vi "PXI_Health_Loop.vi"(8 "error in (no error)":errorcluster) -> (0 "error out":errorcluster)   [LabVIEW 2018]
uses:
  Controls/Enums/PXI_Loop_Enum.ctl
  Controls/Clusts/PXI_Health.ctl
  Controls/Enums/FP_Loop_Enum.ctl
  <vilib>/nisyscfg/Close (Filter).vi
  <vilib>/nisyscfg/Close (Hardware).vi
  <vilib>/nisyscfg/Close (System).vi
  <resource>/objmgr/niflexrioatomicsae.rc
  <vilib>/nisyscfg/nisyscfg.lvlib
panel:
  out "Elapsed (s)":dbl caption="Elapsed Time (s)"
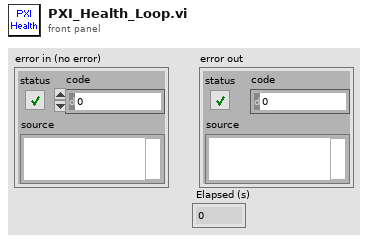
[diagram p1: front panel]
types:
  T1 = typedef "PXI_Loop_Enum.ctl" = enum16{"PXI_Init", "PXI_Time", "PXI_Read", "PXI_Exit"}
  T2 = typedef "PXI_Health.ctl" = cluster{"Temperatures":string[][], "Fans":string[][], "Voltages":string[][]}
  T3 = typedef "FP_Loop_Enum.ctl" = enum16{"FP_Init", "FP_Scale", "FP_Tone", "FP_Noise", "FP_Probes", "FP_PXI", "FP_AI", "FP_TC", "FP_PWR_Hist", "FP_Alarm", "FP_Exit"}
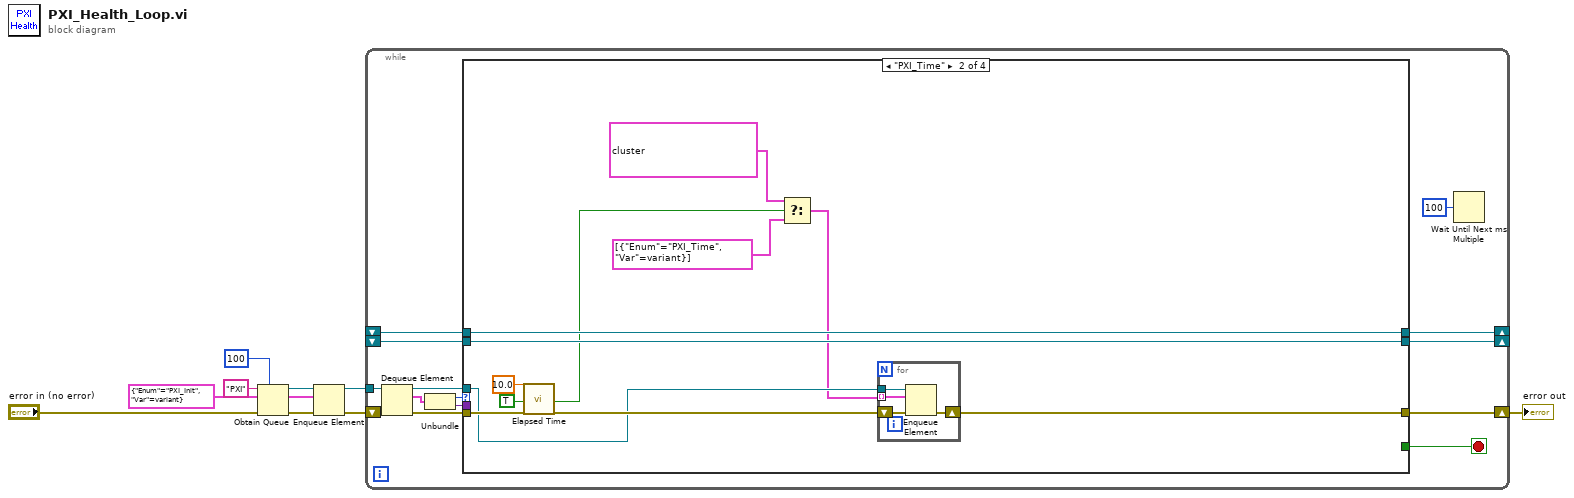
[diagram p0: block diagram]
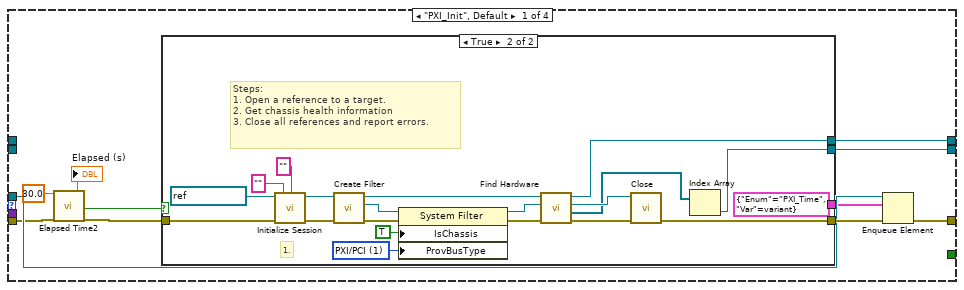
[diagram p2: hidden frame]
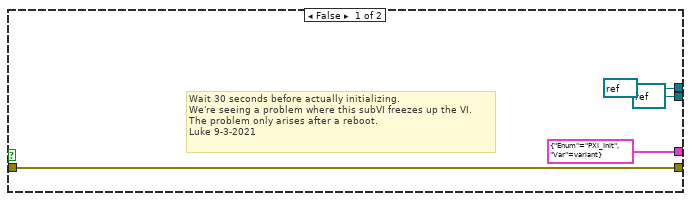
[diagram p3: hidden frame]
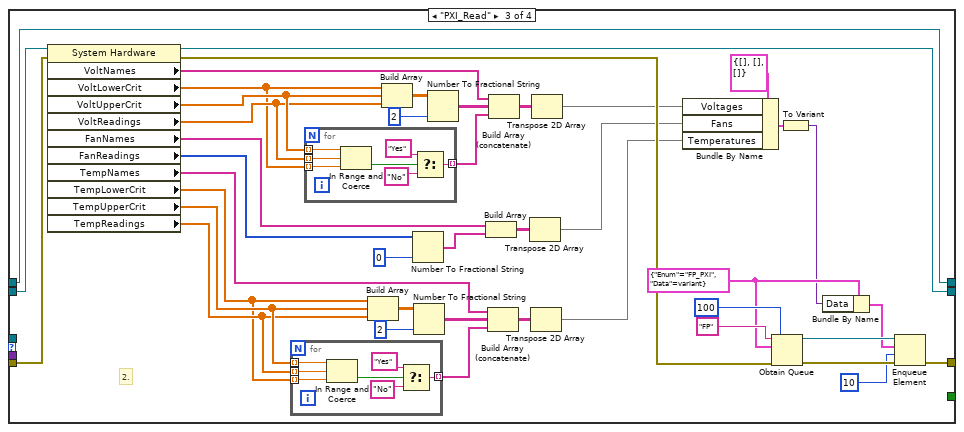
[diagram p4: hidden frame]
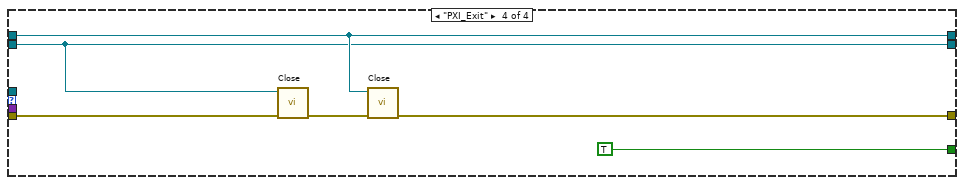
[diagram p5: hidden frame]
diagram:
  w5 = cluster{"Enum":T1, "Var":variant} {"Enum"=enum."PXI_Init", "Var"=variant}
  n1 = Obtain Queue(max queue size (-1, unlimited)=100, name (unnamed)="PXI", element data type=w5, error in (no error)="error in (no error)") -> (queue out=w3:refnum<queue>, error out=w1:errorcluster)  [unwired: 1 in, 1 out]
  n2 = Enqueue Element(queue=w3, element=w5, error in (no error)=w1) -> (queue out=w4:refnum<queue>, error out=w2:errorcluster)  [unwired: 1 in, 1 out]
  n3 = while {
    tunnel: w4 -> [w21]
    shift-right: [w16] -> w8
    shift-left: w2 -> [w22]
    shift-right: [w14] -> _
    shift-left: _ -> [w13]
    shift-right: [w12] -> _
    shift-left: _ -> [w11]
    stop <- w10 stop-if-true
    n4 = Dequeue Element(queue=w21, error in (no error)=w22) -> (queue out=w20:refnum<queue>, element=w18:cluster{"Enum":T1, "Var":variant}, error out=w19:errorcluster)  [unwired: 1 in, 1 out]
    n5 = Unbundle(w18) -> ("Enum"=w15:T1, "Var"=w17:variant)
    n6 = case shown="\"PXI_Time\"" w15 {
      tunnel: w20 -> [w30 w63 _ _]
      tunnel: w19 -> [w27 w70 w92 w135]
      tunnel: w17 -> [_ _ _ _]
      tunnel: [w31 w64 w85 w134] -> w16
      tunnel: [w34 w66 w90 w133] -> w14
      tunnel: w13 -> [_ w66 w90 w133]
      tunnel: [w33 w67 w91 w131] -> w12
      tunnel: w11 -> [_ w67 w93 w131]
      tunnel: [_ _ _ TRUE] -> w10
      frame "PXI_Init", Default {
        n7 = call "Elapsed Time2"("Time Target (s)"=30.0, "error in (no error)"=w27) -> ("Elapsed Time (s)"=→"Elapsed (s)":dbl, "Time has Elapsed"=w25:bool, "error out"=w28:errorcluster)  [unwired: 10 in, 5 out]
        n8 = case shown="True" w25 {
          tunnel: [refnum<k21> refnum ("Session out") w43] -> w34
          tunnel: [refnum<k20> refnum ("resource out") w42] -> w33
          tunnel: [w38 w41] -> w32
          tunnel: [cluster{"Enum":T1, "Var":variant} {"Enum"=enum."PXI_Init", "Var"=variant} ("element") cluster{"Enum":T1, "Var":variant} {"Enum"=enum."PXI_Time", "Var"=variant} ("element")] -> w29
          tunnel: w28 -> [w38 w39]
          frame False {
            # "Wait 30 seconds before actually initializing.\nWe're seeing a problem where this subVI freezes up the VI.\nThe problem only arises after a reboot.\nLuke 9-3-2021"
          }
          frame True {
            w50 = u32 1 items=["BuiltIn/System", "PXI/PCI", "USB", "GPIB", "VXI", "Serial", "TCP/IP", "cRIO", "SCXI", "cDAQ", "SwitchBlock", "SCC"] ("Devices & Chassis:Provides Bus Type")
            # "Steps:\n1. Open a reference to a target.\n2. Get chassis health information\n3. Close all references and report errors."
            # "1."
            n9 = call <vilib>:"Initialize Session.vi"("Password"="", "User Name"="", "error in (no error)"=w39, "Target (localhost)"=refnum<k21> "localhost") -> ("error out"=w48:errorcluster, "Session out"=w49:refnum<k21>)  [unwired: 6 in]
            n10 = call <vilib>:"Create Filter.vi"("error in (no error)"=w48, "Session in"=w49) -> ("error out"=w58:errorcluster, "Filter out"=w55:refnum<k20>, "Session out"=w56:refnum<k21>)  [unwired: 7 in]
            n11 = property class="System Filter"(reference=w55, error in=w58, "IsChassis"=TRUE, "ProvBusType"=w50) -> (reference out=w54:refnum<k20>, error out=w57:errorcluster)
            n12 = call <vilib>:"Find Hardware.vi"("error in (no error)"=w57, "Filter in"=w54, "Session in"=w56) -> ("error out"=w52:errorcluster, "Resources out"=w44:refnum<k20>[], "Filter out"=w53:refnum<k20>, "Session out"=w43:refnum<k21>)  [unwired: 5 in]
            n13 = call-poly <vilib>:"Close.vi"("error in (no error)"=w52, "Filter in"=w53) -> ("error out"=w41:errorcluster)  [unwired: 9 in]
            n14 = Index Array(array=w44) -> (element=w42:refnum<k20>)  [unwired: 1 in]
          }
        }
        n15 = Enqueue Element(queue=w30, element=w29, error in (no error)=w32) -> (error out=w31:errorcluster)  [unwired: 1 in, 2 out]
      }
      frame "PXI_Time" {
        n16 = call "Elapsed Time"("Time Target (s)"=10.0, "Auto Reset"=TRUE, "error in (no error)"=w70) -> ("Time has Elapsed"=w60:bool, "error out"=w65:errorcluster)  [unwired: 9 in, 6 out]
        n17 = Select(t=cluster{"Enum":T1, "Var":variant}[] [{"Enum"=enum."PXI_Read", "Var"=variant}, {"Enum"=enum."PXI_Time", "Var"=variant}], s=w60, f=cluster{"Enum":T1, "Var":variant}[] [{"Enum"=enum."PXI_Time", "Var"=variant}]) -> (s? t:f=w59:cluster{"Enum":T1, "Var":variant}[])
        n18 = for {
          tunnel: w63 -> [w72]
          shift-right: [w73] -> w64
          shift-left: w65 -> [w74]
          tunnel: w59 -> [w71] mode=indexing
          n19 = Enqueue Element(queue=w72, element=w71, error in (no error)=w74) -> (error out=w73:errorcluster)  [unwired: 1 in, 2 out]
        }
      }
      frame "PXI_Read" {
        w83 = cluster{"Enum":T3, "Data":variant} {"Enum"=enum."FP_PXI", "Data"=variant}
        # "2."
        n20 = property class="System Hardware"(reference=w93, error in=w92) -> (reference out=w91:refnum<k20>, error out=w87:errorcluster, "VoltNames"=w114:string[], "VoltLowerCrit"=w110:dbl[], "VoltUpperCrit"=w112:dbl[], "VoltReadings"=w111:dbl[], "FanNames"=w106:string[], "FanReadings"=w105:u32[], "TempNames"=w95:string[], "TempLowerCrit"=w94:dbl[], "TempUpperCrit"=w98:dbl[], "TempReadings"=w97:dbl[])
        n21 = for {
          tunnel: [w120] -> w101 mode=indexing
          tunnel: w98 -> [w119] mode=indexing
          tunnel: w97 -> [w118] mode=indexing
          tunnel: w94 -> [w117] mode=indexing
          n22 = In Range and Coerce(upper limit=w119, x=w118, lower limit=w117) -> (In Range?=w123:bool)  [unwired: 1 out]
          n23 = Select(t="Yes", s=w123, f="No") -> (s? t:f=w120:string)
        }
        n24 = for {
          tunnel: w112 -> [w130] mode=indexing
          tunnel: w111 -> [w129] mode=indexing
          tunnel: w110 -> [w128] mode=indexing
          tunnel: [w124] -> w109 mode=indexing
          n25 = In Range and Coerce(upper limit=w130, x=w129, lower limit=w128) -> (In Range?=w127:bool)  [unwired: 1 out]
          n26 = Select(t="Yes", s=w127, f="No") -> (s? t:f=w124:string)
        }
        n27 = Build Array(w94, w98, w97) -> (w96:dbl[][])
        n28 = Build Array(w110, w112, w111) -> (w116:dbl[][])
        n29 = Number To Fractional String(number=w105, precision (6)=i16 0) -> (F-format string=w104:string[])  [unwired: 2 in]
        n30 = Number To Fractional String(number=w96, precision (6)=i16 2) -> (F-format string=w99:string[][])  [unwired: 2 in]
        n31 = Number To Fractional String(number=w116, precision (6)=i16 2) -> (F-format string=w115:string[][])  [unwired: 2 in]
        n32 = Build Array(w106, w104) -> (w103:string[][])
        n33 = Build Array (concatenate)(w95, w99, w101) -> (w100:string[][])
        n34 = Build Array (concatenate)(w114, w115, w109) -> (w113:string[][])
        n35 = Transpose 2D Array(2D array=w103) -> (transposed array=w79:string[][])
        n36 = Transpose 2D Array(2D array=w100) -> (transposed array=w78:string[][])
        n37 = Transpose 2D Array(2D array=w113) -> (transposed array=w80:string[][])
        n38 = Bundle By Name(cluster=T2 {"Temperatures"=[], "Fans"=[], "Voltages"=[]} ("PXI"), "Voltages"=w80, "Fans"=w79, "Temperatures"=w78) -> (w77:T2)
        n39 = Obtain Queue(max queue size (-1, unlimited)=100, name (unnamed)="FP", element data type=w83, error in (no error)=w87) -> (queue out=w84:refnum<queue>, error out=w86:errorcluster)  [unwired: 1 in, 1 out]
        n40 = To Variant(anything=w77) -> (Variant=w76:variant)
        n41 = Bundle By Name(cluster=w83, "Data"=w76) -> (w82:cluster{"Enum":T3, "Data":variant})
        n42 = Enqueue Element(queue=w84, element=w82, timeout in ms (-1)=10, error in (no error)=w86) -> (error out=w85:errorcluster)  [unwired: 2 out]
      }
      frame "PXI_Exit" {
        n43 = call-poly <vilib>:"Close.vi"("error in (no error)"=w135, "Resource in"=w131) -> ("error out"=w136:errorcluster)  [unwired: 9 in]
        n44 = call-poly <vilib>:"Close.vi"("error in (no error)"=w136, "Session in"=w133) -> ("error out"=w134:errorcluster)  [unwired: 9 in]
      }
    }
    n45 = Wait Until Next ms Multiple(millisecond multiple=u32 100 ("Wait (ms)")) -> ()  [unwired: 1 out]
  }
  "error out" <- w8
